vi "Pockels Cal_Extract relevant cal.vi"(8 "error in (no error)":errorcluster, 9 "Wavelength value":dbl, 11 "Loaded table":string[][](array[string])=[["Cal Wavelength", "", "", ""], ["800", "", "", ""], ["Prism 1:", "2039", "", ""], ["Prism 2:", "2160", "", ""], ["Laser power displayed (mW):", "4000", "", ""], ["Pockels bias:", "199", "", ""], ["Zoom:", "12", "", ""], ["Dwell time:", "0.4", "", ""], ["Cal subset indexes", "", "", ""], ["0", "14", "", ""], ["Cal data", "", "", ""], ["Pockels V", "No objective", "", ""], ["0", "0", "", ""], ["0.1", "5.5", "", ""], ["0.2", "14.5", "", ""], ["0.3", "28.7", "", ""], ["0.4", "47.9", "", ""], ["0.5", "70.6", "", ""], ["0.6", "96.1", "", ""], ["0.7", "123", "", ""], ["0.8", "150", "", ""], ["0.9", "176", "", ""], ["1", "199", "", ""], ["1.1", "219", "", ""], ["1.2", "234", "", ""], ["1.3", "245", "", ""], ["1.4", "249", "", ""], ["1.5", "248", "", ""], ["1.6", "241", "", ""], ["1.7", "228", "", ""], ["1.8", "210", "", ""], ["1.9", "191", "", ""], ["2", "191", "", ""], ["", "", "", ""], ["Cal Wavelength", "", "", ""], ["820", "", "", ""], ["Prism 1:", "2039", "", ""], ["Prism 2:", "1953", "", ""], ["Laser power displayed (mW):", "3960", "", ""], ["Pockels bias:", "199", "", ""], ["Zoom:", "12", "", ""], ["Dwell time:", "0.4", "", ""], ["Cal subset indexes", "", "", ""], ["0", "15", "", ""], ["Cal data", "", "", ""], ["Pockels V", "No objective", "Nikon X", "Nikon 25X"], ["0", "0", "", "0"], ["0.1", "2.8", "", "1.96"], ["0.2", "9.8", "", "6.86"], ["0.3", "21.4", "", "14.98"], ["0.4", "37.1", "", "25.97"], ["0.5", "56.1", "", "39.27"], ["0.6", "77.7", "", "54.39"], ["0.7", "101", "", "70.7"], ["0.8", "125", "", "87.5"], ["0.9", "148", "", "103.6"], ["1", "169", "", "118.3"], ["1.1", "188", "", "131.6"], ["1.2", "204", "", "142.8"], ["1.3", "215", "", "150.5"], ["1.4", "222", "", "155.4"], ["1.5", "225", "", "157.5"], ["1.6", "222", "", "155.4"], ["1.7", "214", "", "149.8"], ["1.8", "202", "", "141.4"], ["1.9", "187", "", "130.9"], ["2", "152", "", "106.4"], ["", "", "", ""], ["Cal Wavelength", "", "", ""], ["850", "", "", ""], ["Prism 1:", "2039", "", ""], ["Prism 2:", "1858", "", ""], ["Laser power displayed (mW):", "3370", "", ""], ["Pockels bias:", "199", "", ""], ["Zoom:", "12", "", ""], ["Dwell time:", "0.4", "", ""], ["Cal subset indexes", "", "", ""], ["0", "15", "", ""], ["Cal data", "", "", ""], ["Pockels V", "No objective", "", ""], ["0", "0", "", ""], ["0.1", "1.2", "", ""], ["0.2", "4.2", "", ""], ["0.3", "8.9", "", ""], ["0.4", "15.1", "", ""], ["0.5", "22.4", "", ""], ["0.6", "30.8", "", ""], ["0.7", "40", "", ""], ["0.8", "49.2", "", ""], ["0.9", "58.3", "", ""], ["1", "66.7", "", ""], ["1.1", "74.6", "", ""], ["1.2", "81", "", ""], ["1.3", "86", "", ""], ["1.4", "89.6", "", ""], ["1.5", "90.9", "", ""], ["1.6", "90.5", "", ""], ["1.7", "88.3", "", ""], ["1.8", "84.1", "", ""], ["1.9", "79.5", "", ""], ["2", "79.3", "", ""], ["", "", "", ""], ["Cal Wavelength", "", "", ""], ["920", "", "", ""], ["Prism 1:", "2039", "", ""], ["Prism 2:", "1096", "", ""], ["Laser power displayed (mW):", "2100", "", ""], ["Pockels bias:", "199", "", ""], ["Zoom:", "12", "", ""], ["Dwell time:", "0.4", "", ""], ["Cal subset indexes", "", "", ""], ["0", "15", "", ""], ["Cal data", "", "", ""], ["Pockels V", "No objective", "", ""], ["0", "0", "", ""], ["0.1", "6.3", "", ""], ["0.2", "11", "", ""], ["0.3", "16.7", "", ""], ["0.4", "23.5", "", ""], ["0.5", "31", "", ""], ["0.6", "38.8", "", ""], ["0.7", "47", "", ""], ["0.8", "54.9", "", ""], ["0.9", "62.5", "", ""], ["1", "69.3", "", ""], ["1.1", "75.3", "", ""], ["1.2", "80", "", ""], ["1.3", "83.5", "", ""], ["1.4", "85.2", "", ""], ["1.5", "85.6", "", ""], ["1.6", "84.6", "", ""], ["1.7", "82.2", "", ""], ["1.8", "78.5", "", ""], ["1.9", "73.7", "", ""], ["2", "73.7", "", ""]]) -> (0 "error out":errorcluster, 1 "Index of replacement":i32, 2 "Multiplier for power after the objective":dbl, 3 "Relevant cal only":string[][](array[string]))   [LabVIEW 2013]
uses:
  Program Files (x86)/National Instruments/LabVIEW 2013/user.lib/_OpenG.lib/array/array.llb/Search 1D Array (String)__ogtk.vi
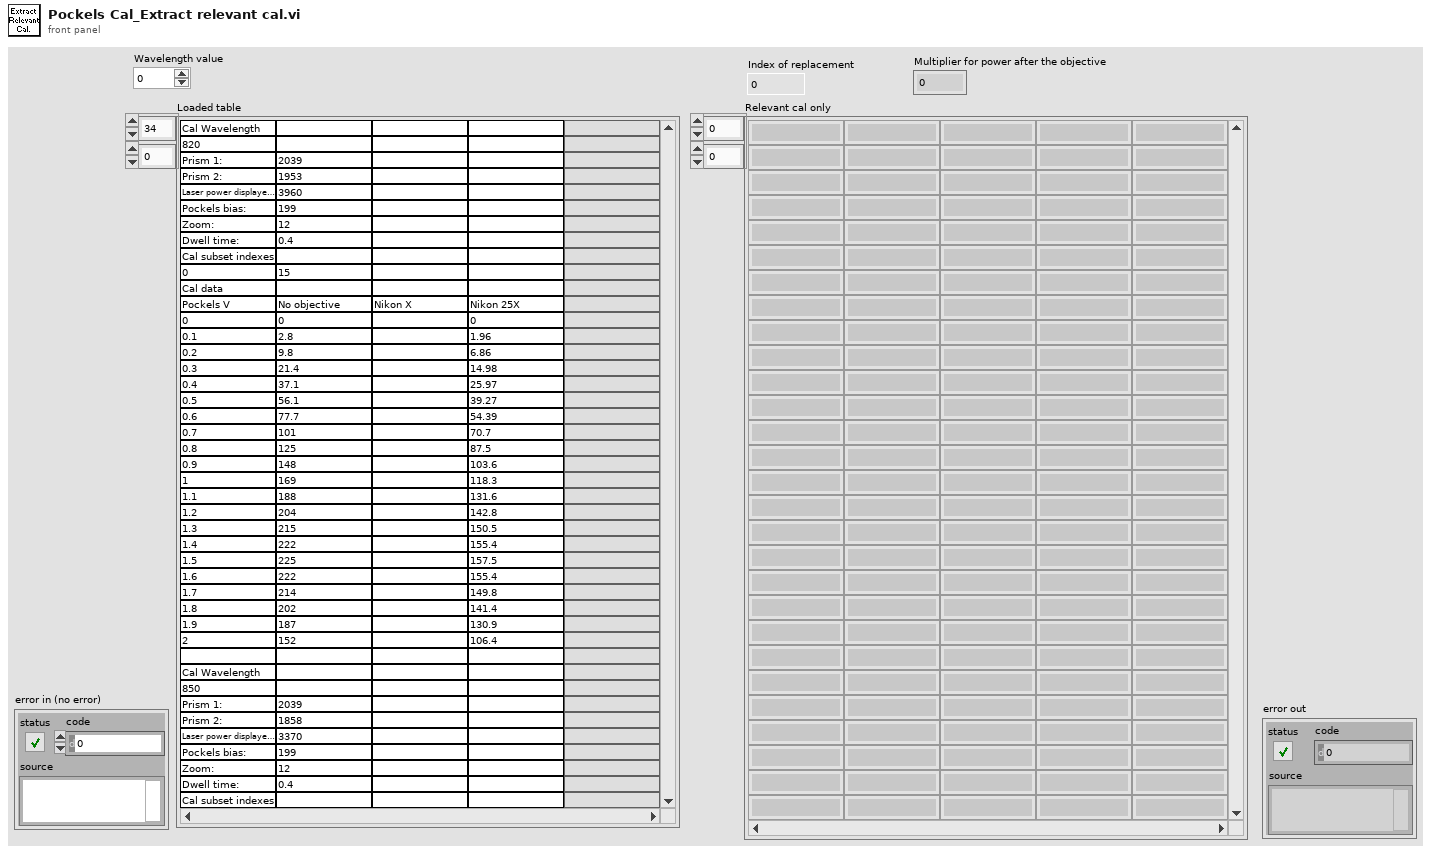
[diagram p1: front panel]
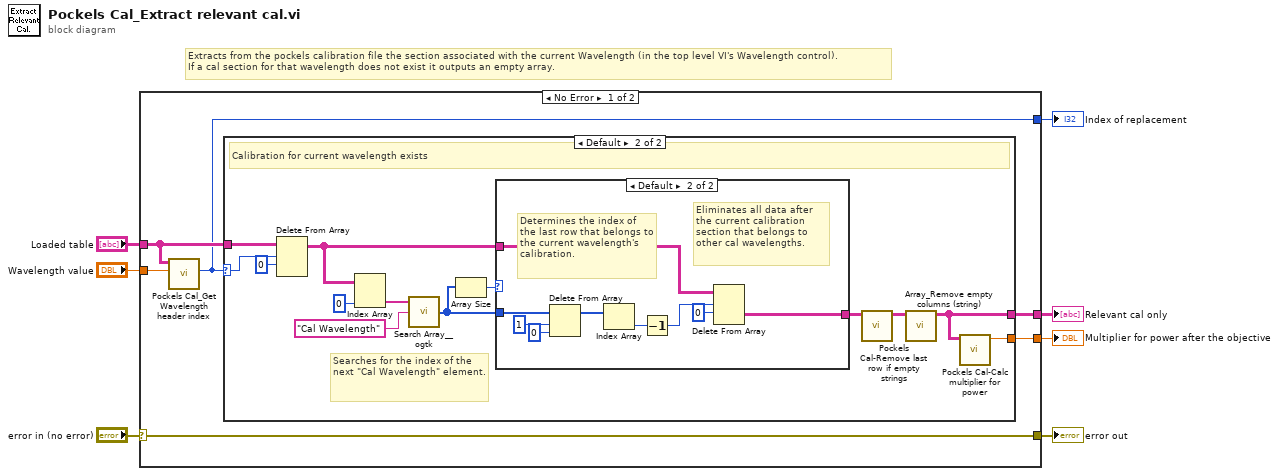
[diagram p0: block diagram]
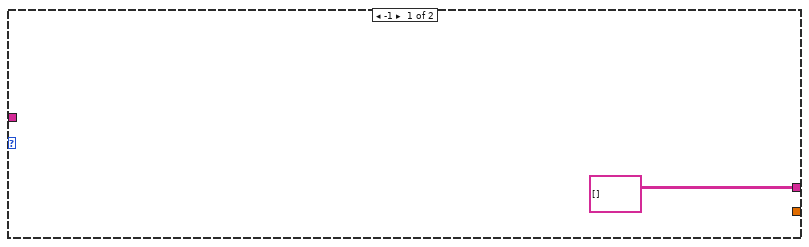
[diagram p2: hidden frame]
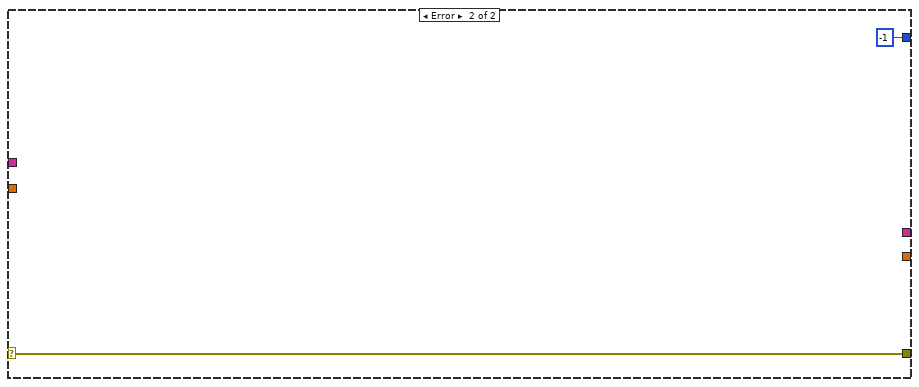
[diagram p4: hidden frame]
diagram:
  # "Extracts from the pockels calibration file the section associated with the current Wavelength (in the top level VI's Wavelength control).\nIf a cal section for that wavelength does not exist it outputs an empty array."
  n1 = case shown="No Error" "error in (no error)" {
    selector: "error in (no error)" -> [w9 w39]
    tunnel: "Loaded table" -> [w13 _]
    tunnel: [w12 _] -> w6
    tunnel: [w11 -1 ("Index of \"Cal Wavelength\" header")] -> w5
    tunnel: "Wavelength value" -> [w10 _]
    tunnel: [w9 w39] -> w2
    tunnel: [w8 _] -> w1
    frame No Error {
      n2 = call "Pockels Cal_Get Wavelength header index.vi"("Waveform"=w10, "Loaded cal file"=w13) -> ("Index of \"Cal Wavelength\" header"=w11:i32)  [unwired: 8 in, 1 out]
      n3 = case shown="Default" w11 {
        selector: w11 -> [_ w19]
        tunnel: w13 -> [_ w23]
        tunnel: [string[][] [] ("Loaded table") w15] -> w12
        tunnel: [_ w18] -> w8
        frame -1 {
        }
        frame Default {
          # "Searches for the index of the next \"Cal Wavelength\" element."
          # "Calibration for current wavelength exists"
          n4 = Delete From Array "Delete From Array"(array=w23, length=w19, index (row)=0) -> (array with subset deleted=w22:string[][])  [unwired: 1 in, 1 out]
          n5 = Index Array "Index Array"(array=w22, index (col)=0 ("disabled index (col)")) -> (element=w25:string[])  [unwired: 1 in]
          n6 = call-poly "Search Array__ogtk.vi"("Array"=w25, "Element Data"="Cal Wavelength" ("element")) -> ("Indices of Elements"=w20:i32[])  [unwired: 7 in]
          n7 = Array Size(array=w20) -> (size(s)=w21:i32)
          n8 = case shown="Default" w21 {
            tunnel: w20 -> [_ w36]
            tunnel: w22 -> [w28 w32]
            tunnel: [w28 w31] -> w17
            frame 0, 1 {
              # "No additional calibration sections exist after\nthe one of interest."
            }
            frame Default {
              # "Eliminates all data after the current calibration section that belongs to other cal wavelengths."
              # "Determines the index of the last row that belongs to the current wavelength's calibration."
              n9 = Delete From Array "Delete From Array"(array=w36, length=1, index=0) -> (array with subset deleted=w33:i32[])  [unwired: 1 out]
              n10 = Index Array(array=w33) -> (element=w30:i32)  [unwired: 1 in]
              n11 = Decrement(x=w30) -> (x-1=w29:i32)
              n12 = Delete From Array "Delete From Array"(array=w32, length=w29, index (row)=0) -> (deleted portion=w31:string[][])  [unwired: 1 in, 1 out]
            }
          }
          n13 = call "Pockels Cal-Remove last row if empty strings.vi"("Pockels Cal table"=w17) -> ("Pockels Cal table (inc. header line)"=w16:string[][])  [unwired: 10 in]
          n14 = call "Array_Remove empty columns (string).vi"("Pockels Cal table"=w16) -> ("Pockels Cal table (inc. header line)"=w15:string[][])  [unwired: 10 in]
          n15 = call "Pockels Cal-Calc multiplier for power.vi"("Pockels Cal table"=w15) -> ("Multiplier for power after the objective"=w18:dbl)  [unwired: 10 in]
        }
      }
    }
    frame Error {
    }
  }
  "Relevant cal only" <- w6
  "Index of replacement" <- w5
  "error out" <- w2
  "Multiplier for power after the objective" <- w1
